vi "ActionVIOnDelete.vi"(6 "All deleted Refs":T1[](array[typedef]) format="%.0x", 8 "error in (no error)":errorcluster, 11 "Item Ref in":T1 format="%.0x") -> (0 "error out":errorcluster, 3 "Item Ref out":T1 format="%.0x")   [LabVIEW 2019, in "Diagnostics Addon System Explorer.lvlib"]
uses:
  Diagnostics Addon System Explorer.lvlib
  <vilib>/NI VeriStand/Custom Device API/Custom Device Item Ref.ctl
  Shared/SubVIs/Constants.vi
  <vilib>/NI VeriStand/Custom Device Tools/Custom Device Utility Library/NI VeriStand - Search for All Items by GUID.vi
  <vilib>/NI VeriStand/Custom Device Tools/Custom Device Utility Library/NI VeriStand - Search for Item by GUID.vi
  <vilib>/NI VeriStand/Custom Device Tools/Custom Device Utility Library/NI VeriStand - Search for Item by Name.vi
  <vilib>/NI VeriStand/Custom Device Tools/Custom Device Utility Library/Custom Device Utility Library.lvlib
  Shared/Diagnostics Addon Shared.lvlib
  <vilib>/NI VeriStand/Custom Device API/Custom Device API.lvlib
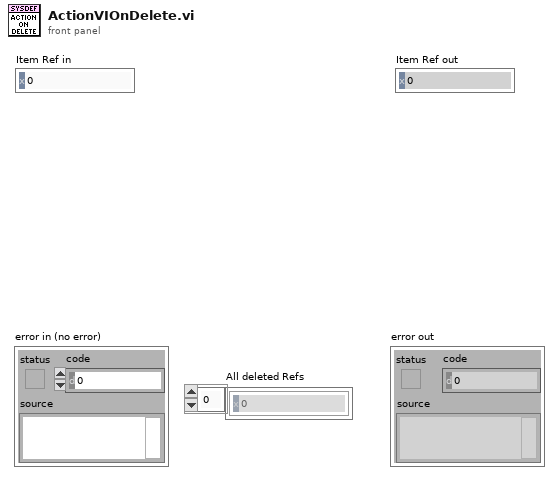
[diagram p1: front panel]
types:
  T1 = typedef "Custom Device API.lvlib/Custom Device Item Ref.ctl" = u64
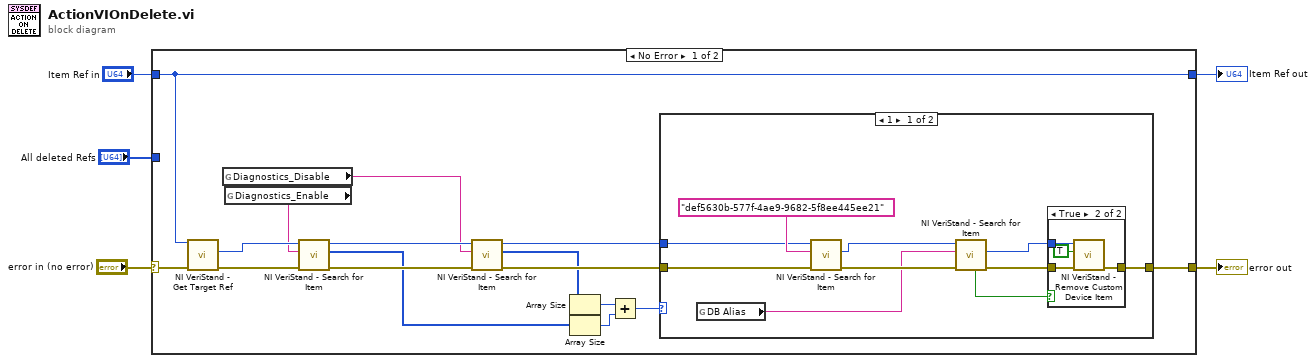
[diagram p0: block diagram]
diagram:
  n1 = case shown="No Error" "error in (no error)" {
    selector: "error in (no error)" -> [w20 w39]
    tunnel: [w12 w39] -> w4
    tunnel: "Item Ref in" -> [w21 w38]
    tunnel: [w21 w38] -> w2
    tunnel: "All deleted Refs" -> [_ _]
    frame No Error {
      n2 = call <vilib>:"NI VeriStand - Get Target Ref.vi"("error in"=w20, "Item Ref in"=w21) -> ("error out"=w18:errorcluster, "Target Ref"=w19:T1)  [unwired: 6 in, 2 out]
      n3 = global read "Constants.vi" "Diagnostics_Disable"() -> (w14:string)
      n4 = global read "Constants.vi" "Diagnostics_Enable"() -> (w17:string)
      n5 = call-poly <vilib>:"NI VeriStand - Search for Item.vi"("error in"=w18, "Item GUID"=w17, "Section Ref in"=w19) -> ("error out"=w15:errorcluster, "Item Refs"=w10:T1[], "Section Ref out"=w16:T1)  [unwired: 5 in, 1 out]
      n6 = call-poly <vilib>:"NI VeriStand - Search for Item.vi"("error in"=w15, "Item GUID"=w14, "Section Ref in"=w16) -> ("error out"=w13:errorcluster, "Item Refs"=w9:T1[], "Section Ref out"=w11:T1)  [unwired: 5 in, 1 out]
      n7 = Array Size(array=w9) -> (size(s)=w8:i32)
      n8 = Array Size(array=w10) -> (size(s)=w7:i32)
      n9 = Add(x=w8, y=w7) -> (x+y=w6:i32)
      n10 = case shown="1" w6 {
        tunnel: w13 -> [w30 w37]
        tunnel: [w24 w37] -> w12
        tunnel: w11 -> [w23 _]
        frame 1 {
          n11 = global read "Constants.vi" "DB Alias"() -> (w27:string)
          n12 = call-poly <vilib>:"NI VeriStand - Search for Item.vi"("error in"=w30, "Item GUID"="def5630b-577f-4ae9-9682-5f8ee445ee21" ("string"), "Section Ref in"=w23) -> ("error out"=w28:errorcluster, "Item Ref"=w29:T1)  [unwired: 5 in, 2 out]
          n13 = call-poly <vilib>:"NI VeriStand - Search for Item.vi"("error in"=w28, "Item Name"=w27, "Section Ref in"=w29) -> ("error out"=w25:errorcluster, "Item Ref"=w26:T1, "Found"=w22:bool)  [unwired: 5 in, 1 out]
          n14 = case shown="True" w22 {
            tunnel: w26 -> [_ w36]
            tunnel: w25 -> [w32 w35]
            tunnel: [w32 w34] -> w24
            frame False {
            }
            frame True {
              n15 = call <vilib>:"NI VeriStand - Remove Custom Device Item.vi"("error in (no error)"=w35, "Force Delete (F)"=TRUE, "Item Ref in"=w36) -> ("error out"=w34:errorcluster)  [unwired: 7 in, 1 out]
            }
          }
        }
        frame Default {
        }
      }
    }
    frame Error {
    }
  }
  "error out" <- w4
  "Item Ref out" <- w2
